vi "Create-element.vi"(8 "error in (no error)":errorcluster, 10 "String in":string) -> (0 "error out":errorcluster, 1 "Start tag?":bool, 2 "Remaining string":string, 3 "Element-XML out":refnum<class "Element-XML.lvclass">)   [LabVIEW 2013, in "MaterialCharacterization.lvlib" / "Element-XML.lvclass"]
uses:
  Element-XML.lvclass
  Elements.ctl
  WriteDigital/WriteDigital.lvclass
  WriteAnalog/WriteAnalog.lvclass
  Set/Set.lvclass
  ApplicationEvent/ApplicationEvent.lvclass
  JumpAbs/JumpAbs.lvclass
  MarkAbs/MarkAbs.lvclass
  JumpRel/JumpRel.lvclass
  MarkRel/MarkRel.lvclass
  BeginJob/BeginJob.lvclass
  EndJob/EndJob.lvclass
  LongDelay/LongDelay.lvclass
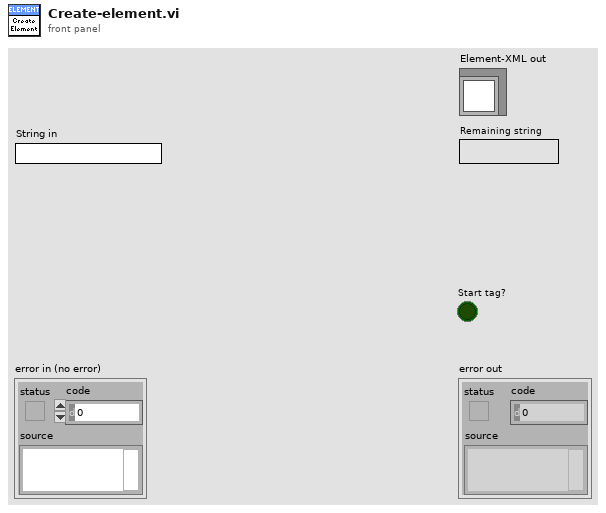
[diagram p1: front panel]
types:
  T1 = typedef "MaterialCharacterization.lvlib/Element-XML.lvclass/Elements.ctl" = enum16{"BeginJob", "WriteDigital", "WriteAnalog", "Set", "ApplicationEvent", "JumpAbs", "MarkAbs", "JumpRel", "MarkRel", "LongDelay", "EndJob"}
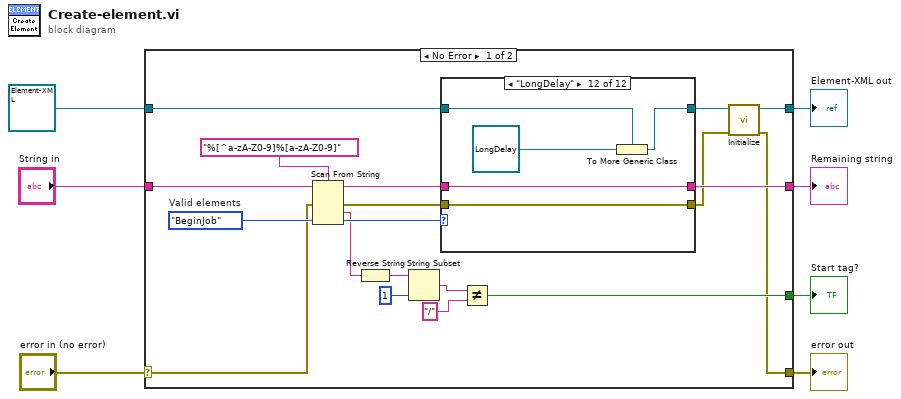
[diagram p0: block diagram]
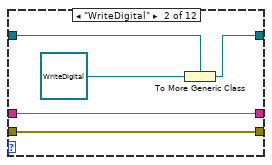
[diagram p3: hidden frame]
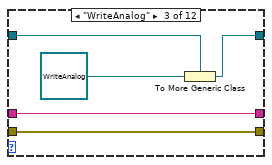
[diagram p4: hidden frame]
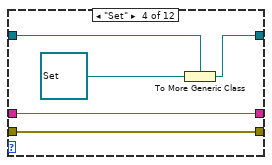
[diagram p5: hidden frame]
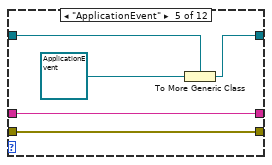
[diagram p6: hidden frame]
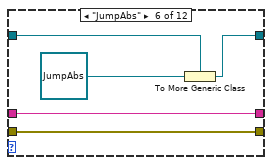
[diagram p7: hidden frame]
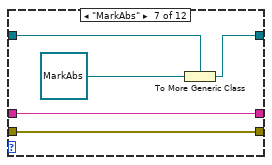
[diagram p8: hidden frame]
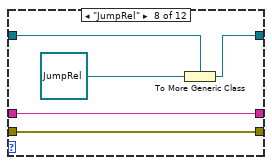
[diagram p9: hidden frame]
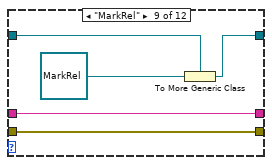
[diagram p10: hidden frame]
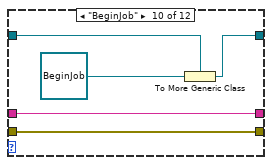
[diagram p11: hidden frame]
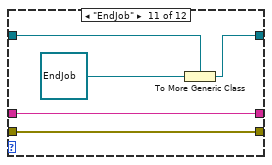
[diagram p12: hidden frame]
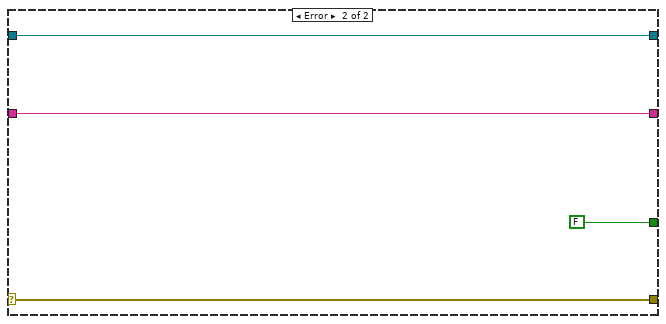
[diagram p13: hidden frame]
diagram:
  n1 = case shown="No Error" "error in (no error)" {
    selector: "error in (no error)" -> [w14 w88]
    tunnel: [w8 w88] -> w6
    tunnel: [w10 w87] -> w4
    tunnel: refnum<class "Element-XML.lvclass"> refnum ("Element-XML in") -> [w24 w87]
    tunnel: "String in" -> [w26 w85]
    tunnel: [w15 FALSE] -> w2
    tunnel: [w12 w85] -> w1
    frame No Error {
      w21 = Elements."BeginJob"  # Valid elements
      n2 = Scan From String(format string="%[^a-zA-Z0-9]%[a-zA-Z0-9]", input string=w26, error in=w14, default 2=w21) -> (remaining string=w13:string, error out=w23:errorcluster, output 1=w19:string, output 2=w22:T1)  [unwired: 2 in, 1 out]
      n3 = Reverse String(1:w19) -> (0:w20:string)
      n4 = String Subset(string=w20, length (rest)=1 ("length (rest)")) -> (substring=w17:string)  [unwired: 1 in]
      n5 = case shown="\"LongDelay\"" w22 {
        tunnel: w24 -> [w29 w32 w38 w43 w48 w53 w58 w63 w68 w73 w78 w83]
        tunnel: w23 -> [w28 w31 w37 w42 w47 w52 w57 w62 w67 w72 w77 w82]
        tunnel: [w29 w33 w39 w44 w49 w54 w59 w64 w69 w74 w79 w84] -> w11
        tunnel: [w28 w31 w37 w42 w47 w52 w57 w62 w67 w72 w77 w82] -> w9
        tunnel: w13 -> [w27 w30 w35 w40 w45 w50 w55 w60 w65 w70 w75 w80]
        tunnel: [w27 w30 w35 w40 w45 w50 w55 w60 w65 w70 w75 w80] -> w12
        frame Default {
        }
        frame "WriteDigital" {
          n6 = To More Generic Class(target class=w32, reference=refnum<class "WriteDigital.lvclass"> refnum ("WriteDigital.lvclass")) -> (generic class reference=w33:refnum<class "Element-XML.lvclass">)
        }
        frame "WriteAnalog" {
          n7 = To More Generic Class(target class=w38, reference=refnum<class "WriteAnalog.lvclass"> refnum ("WriteAnalog.lvclass")) -> (generic class reference=w39:refnum<class "Element-XML.lvclass">)
        }
        frame "Set" {
          n8 = To More Generic Class(target class=w43, reference=refnum<class "Set.lvclass"> refnum ("Set.lvclass")) -> (generic class reference=w44:refnum<class "Element-XML.lvclass">)
        }
        frame "ApplicationEvent" {
          n9 = To More Generic Class(target class=w48, reference=refnum<class "ApplicationEvent.lvclass"> refnum ("ApplicationEvent.lvclass")) -> (generic class reference=w49:refnum<class "Element-XML.lvclass">)
        }
        frame "JumpAbs" {
          n10 = To More Generic Class(target class=w53, reference=refnum<class "JumpAbs.lvclass"> refnum ("JumpAbs.lvclass")) -> (generic class reference=w54:refnum<class "Element-XML.lvclass">)
        }
        frame "MarkAbs" {
          n11 = To More Generic Class(target class=w58, reference=refnum<class "MarkAbs.lvclass"> refnum ("MarkAbs.lvclass")) -> (generic class reference=w59:refnum<class "Element-XML.lvclass">)
        }
        frame "JumpRel" {
          n12 = To More Generic Class(target class=w63, reference=refnum<class "JumpRel.lvclass"> refnum ("MarkAbs.lvclass")) -> (generic class reference=w64:refnum<class "Element-XML.lvclass">)
        }
        frame "MarkRel" {
          n13 = To More Generic Class(target class=w68, reference=refnum<class "MarkRel.lvclass"> refnum ("MarkAbs.lvclass")) -> (generic class reference=w69:refnum<class "Element-XML.lvclass">)
        }
        frame "BeginJob" {
          n14 = To More Generic Class(target class=w73, reference=refnum<class "BeginJob.lvclass"> refnum ("MarkAbs.lvclass")) -> (generic class reference=w74:refnum<class "Element-XML.lvclass">)
        }
        frame "EndJob" {
          n15 = To More Generic Class(target class=w78, reference=refnum<class "EndJob.lvclass"> refnum ("MarkAbs.lvclass")) -> (generic class reference=w79:refnum<class "Element-XML.lvclass">)
        }
        frame "LongDelay" {
          n16 = To More Generic Class(target class=w83, reference=refnum<class "LongDelay.lvclass"> refnum ("MarkAbs.lvclass")) -> (generic class reference=w84:refnum<class "Element-XML.lvclass">)
        }
      }
      n17 = Not Equal?(x=w17, y="/") -> (x != y?=w15:bool)
      n18 = call-dynamic "Initialize.vi"("error in (no error)"=w9, "Element-XML in"=w11) -> ("error out"=w8:errorcluster, "Element-XML out"=w10:refnum<class "Element-XML.lvclass">)  [unwired: 8 in]
    }
    frame Error {
    }
  }
  "error out" <- w6
  "Element-XML out" <- w4
  "Start tag?" <- w2
  "Remaining string" <- w1
